vi "Byte Array to Boolean.vi"(6 "Data 5":u8, 7 "Data 4":u8, 8 "Data 3":u8, 9 "Data 2":u8, 10 "Data 1":u8, 11 "Data 0":u8) -> (0 "In3":bool, 1 "In2":bool, 2 "In1":bool, 3 "In0":bool, 4 "In5":bool, 5 "In4":bool)   [LabVIEW 2015]
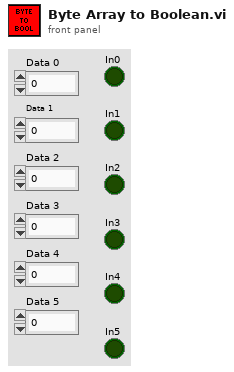
[diagram p1: front panel]
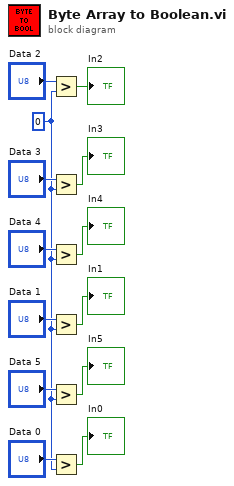
[diagram p0: block diagram]
diagram:
  w7 = u8 0
  n1 = Greater?(x="Data 2", y=w7) -> (0:→"In2":bool)
  n2 = Greater?(x="Data 3", y=w7) -> (0:→"In3":bool)
  n3 = Greater?(x="Data 4", y=w7) -> (0:→"In4":bool)
  n4 = Greater?(x="Data 1", y=w7) -> (0:→"In1":bool)
  n5 = Greater?(x="Data 5", y=w7) -> (0:→"In5":bool)
  n6 = Greater?(x="Data 0", y=w7) -> (0:→"In0":bool)
